vi "Validate Variable Header.vi"(8 "error in (no error)":errorcluster, 11 "ControlPacket in":refnum<class "ControlPacket.lvclass">) -> (0 "error out":errorcluster, 1 "valid?":bool, 3 "ControlPacket out":refnum<class "ControlPacket.lvclass">)   [LabVIEW 2013, in "MQTT_Control_Packets.lvlib" / "ControlPacket.lvclass"]
uses:
  ControlPacket.lvclass
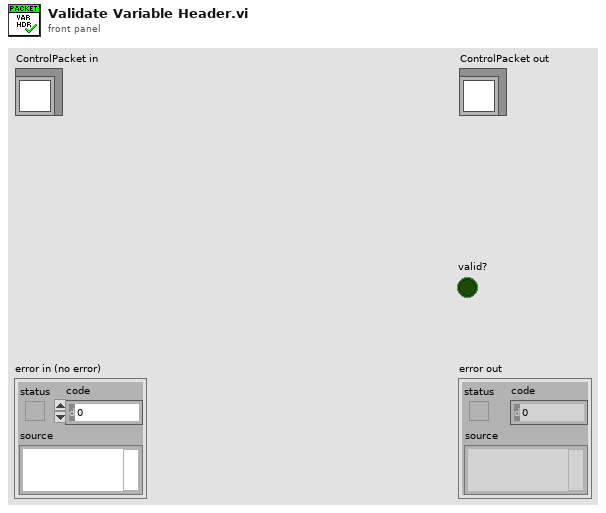
[diagram p1: front panel]
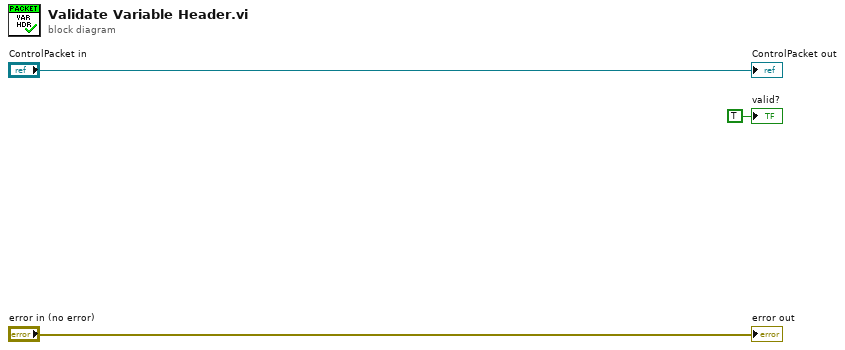
[diagram p0: block diagram]
diagram:
  "error out" <- "error in (no error)"
  "ControlPacket out" <- "ControlPacket in"
  "valid?" <- TRUE ("valid?")
